vi "Set Current Directory.vi"(8 "error in (no error)":errorcluster, 11 "Path":path) -> (0 "error out":errorcluster)   [LabVIEW 2015, in "Win32 Util.lvlib"]
uses:
  Win32 Util.lvlib
  kernel32.dll
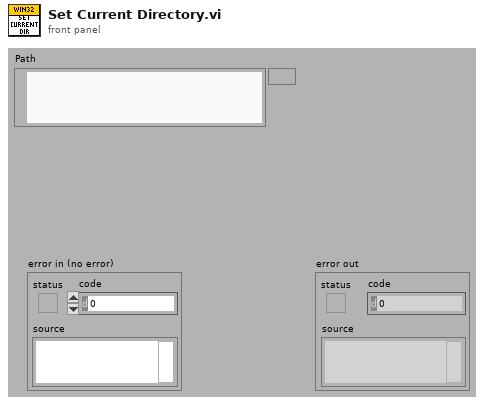
[diagram p1: front panel]
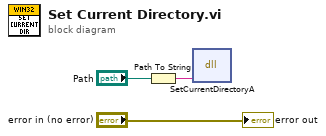
[diagram p0: block diagram]
diagram:
  n1 = Path To String(path="Path") -> (string=w2:string)
  n2 = dll-call lib="kernel32.dll" fn="SetCurrentDirectoryA" label="GetCurrentDirectory"("Directory"=w2) -> ()  [unwired: 4 in, 3 out]
  "error out" <- "error in (no error)"
